vi "input into database.vi"() -> ()   [LabVIEW 2016]
uses:
  controls/db cluster.ctl
  <vilib>/addons/database/Connection.llb/DB Tools Open Connec (String).vi
  <vilib>/Utility/file.llb/Read From Spreadsheet File (string).vi
  <vilib>/addons/database/NI_Database_API.lvlib
panel:
  in  "runnumber":string
  out "output cluster 2":T1
  out "error out":errorcluster
  out "error out 2":errorcluster
  out "element":string="{0.023339,0.023338,0.023336,0.023338,0.023336,0.023336,0.023334\r\n}"
  out "readouts string":string="\r\n1/4/2012 10:09:06 AM\t103752\tWeavCaMB11\tb\tJackson\t0\t3\t50\t1231.000000\tInf\t35.314700\t5.667000\t336.000000\t0.988235\t3599.788248\t31.964787\t6135967.567040\t26573.858939\t1411896.374545\t0.000620\t59.996471\t23532.990455\tNaN\tInf\t0.000000\tNaN\t0.000000\t879579.012026\tNaN\t26573.858939\t0.433083\tNaN\tNaN\tNaN\t7.758172"
  in  "beamline readbacks":T2={"Injector"=[0.023339, 0.023338, 0.023336000000000003, 0.023338, 0.023336000000000003, 0.023336000000000003, 0.023334], "Analyze"=[0.0058, 0.0058, 0.0058, 0.0058, 0.0058, 0.0058, 0.0058], "Switch"=[0.0, 0.0, 0.0, 0.0, 0.0, 0.0, 0.0], "Terminal"=[0.0010328292846679688, 0.0010328292846679688, 0.0013613700866699219, 0.0007047653198242188, 0.0010328292846679688, 0.0010328292846679688, 0.0010328292846679688], "Cathode"=[10.239062309265137, 10.239218711853027, 10.239218711853027, 10.239218711853027, 10.239218711853027, 10.239218711853027, 10.239218711853027]}
  out "db cluster":T3={"startat"="\r\n1/4/2012 10:09:06 AM", "holderid"="103752", "Sample Name"="WeavCaMB11", "type"="b", "User Name"="Jackson", "cycle measured"="0", "position"="3", "estimated ratio"="50", "cycle"="1231.000000", "Transmission"="Inf", "first currents"="35.314700", "runtime"="5.667000", "total rare counts"="336.000000", "livetime"="0.988235", "Rare CPM"="3599.788248", "second current"="31.964787", "17O ratio"="6135967.567040", "17O error"="26573.858939", "Cycle Ratio"="1411896.374545", "cycle error"="0.000620", "interference"="59.996471", "use"="True", "InjSS"="NaN", "He SS"="Inf", "Oaverage"="0.000000", "wheelnumber"="46", "wheel name"="cycle results testdbrunorder.txt", "runnumber"="{0.023339,0.023338,0.023336,0.023338,0.023336,0.023336,0.023334\r\n}", "runletter"="{0.005800,0.005800,0.005800,0.005800,0.005800,0.005800,0.005800\r\n}", "runletter 2"="{0.000000,0.000000,0.000000,0.000000,0.000000,0.000000,0.000000\r\n}"}
  out "name 2":string
  out "name":string
  in  "beamline readbacks 2":T2
  in  "Wheel Number":string
  in  "runletter":string
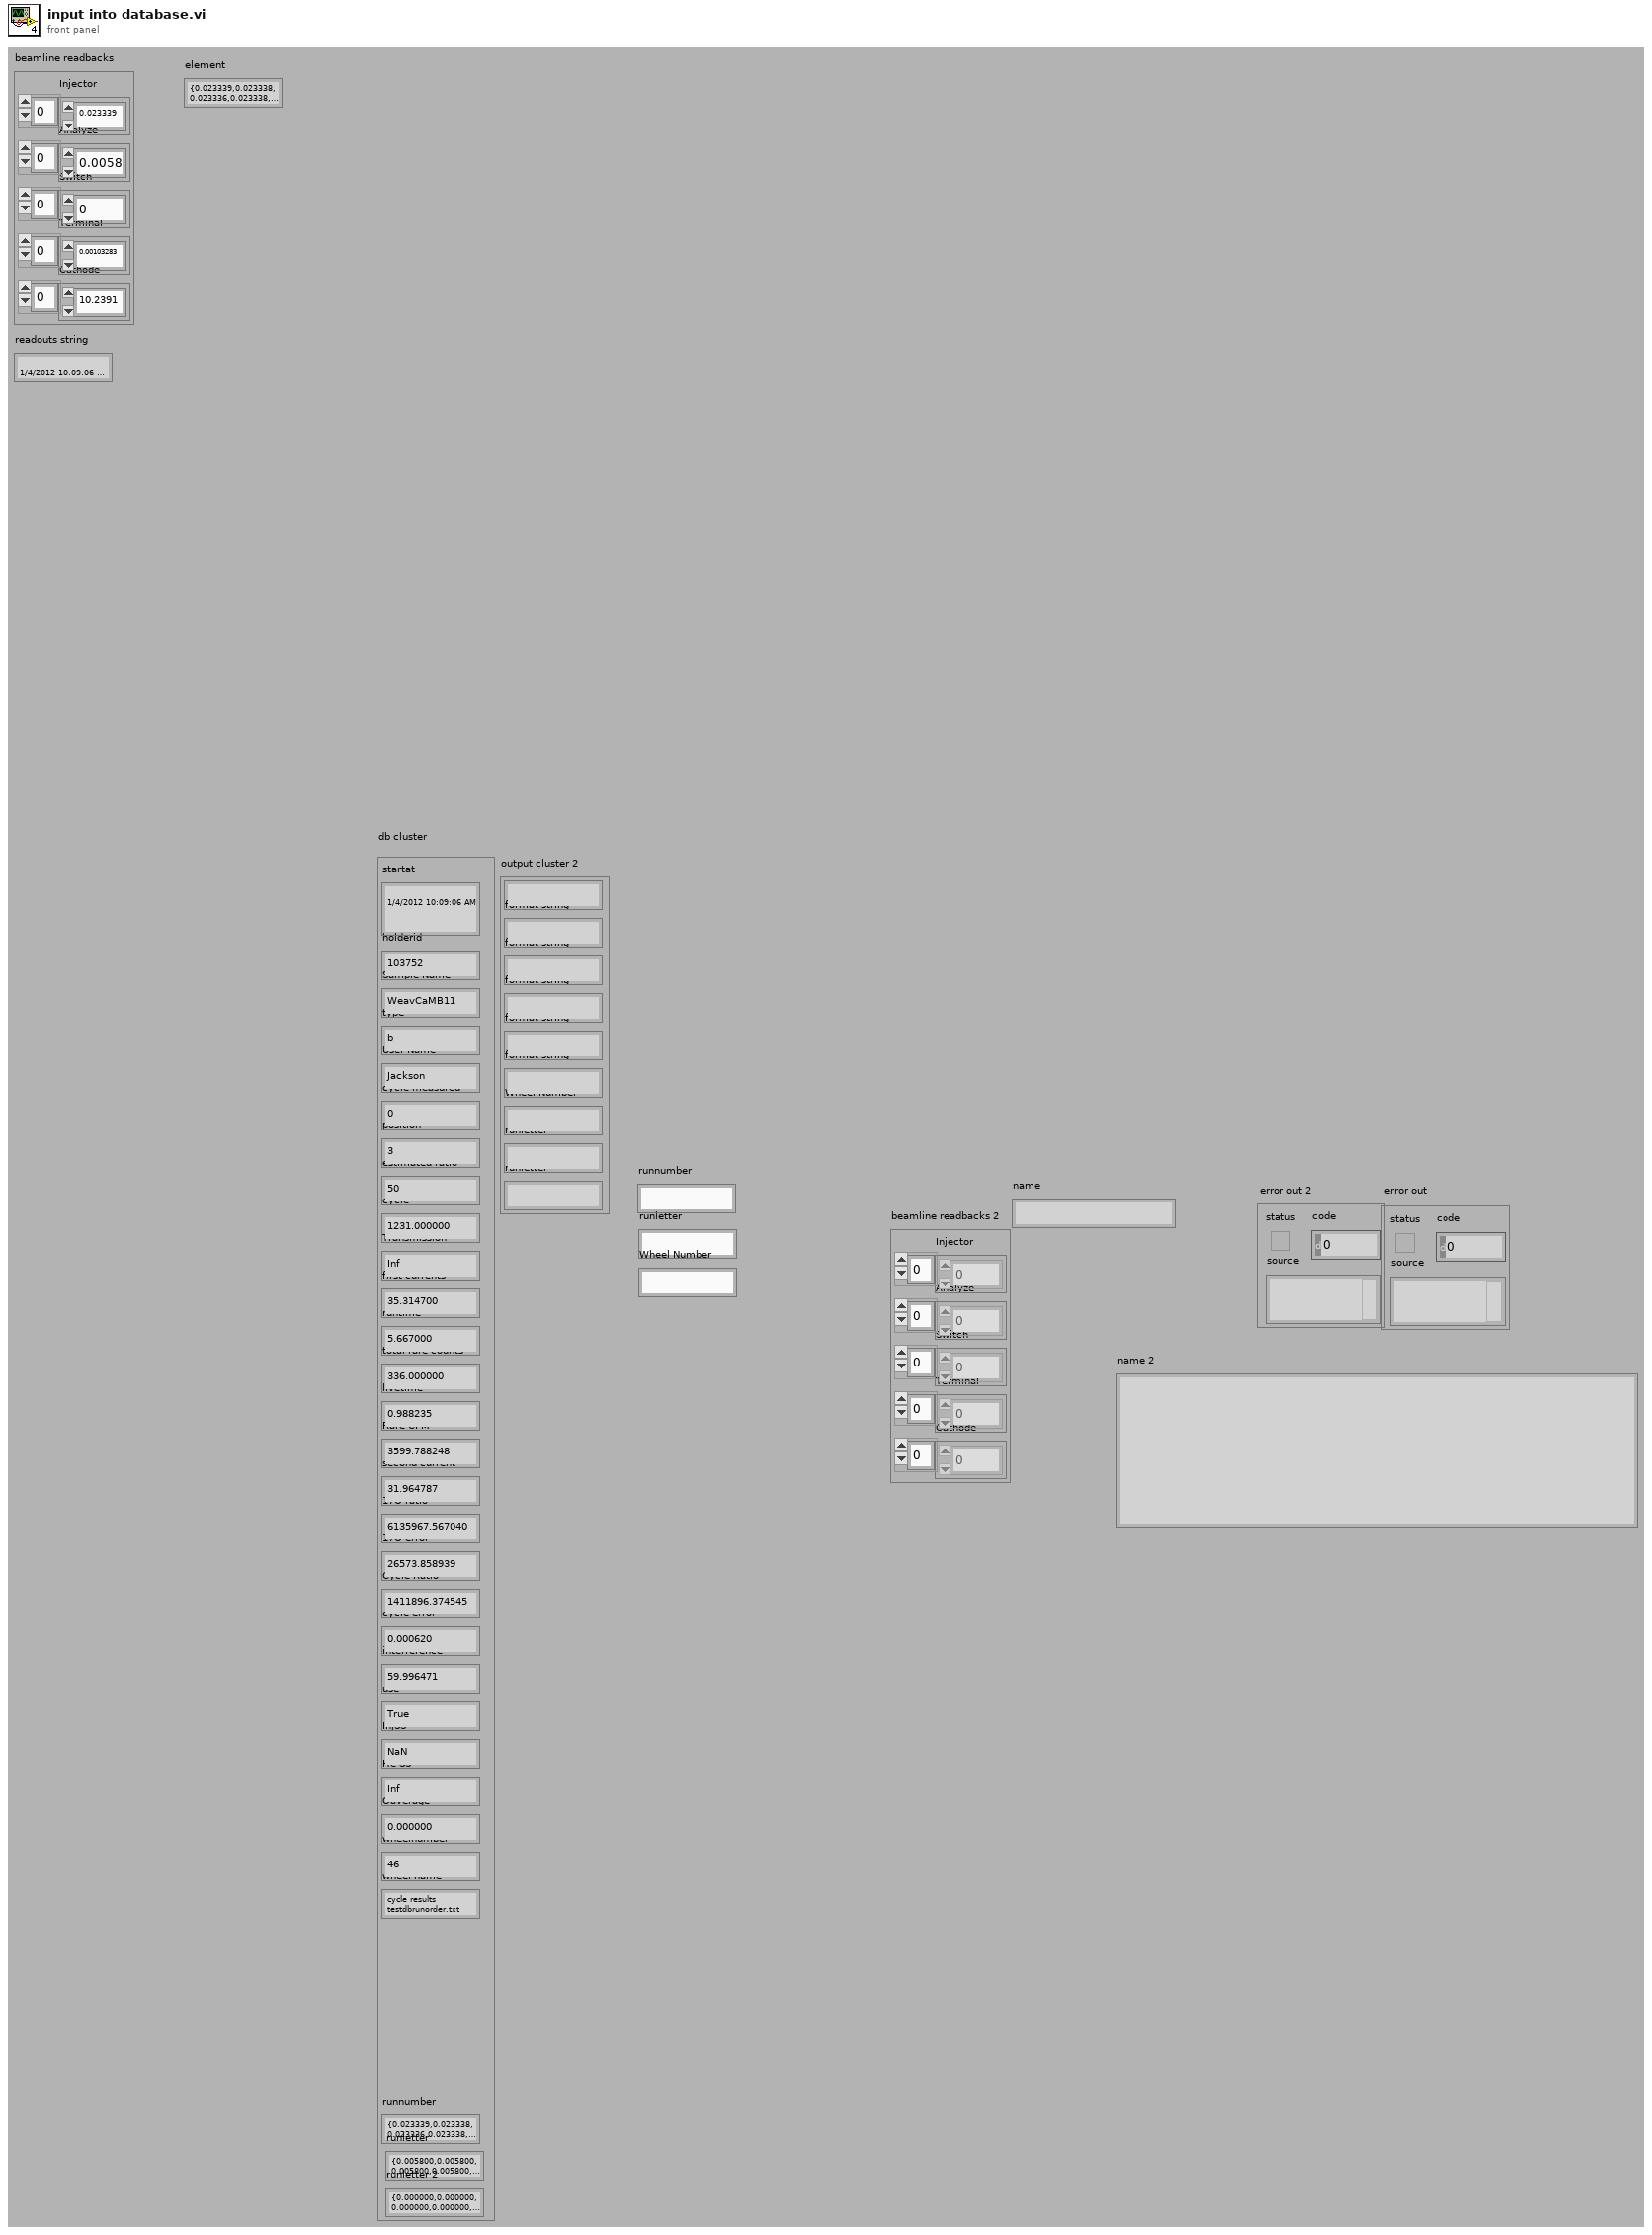
[diagram p1: front panel]
types:
  T1 = cluster{string, "format string":string, "format string":string, "format string":string, "format string":string, "format string":string, "Wheel Number":string, "runletter":string, "runletter":string}
  T2 = cluster{"Injector":dbl[], "Analyze":dbl[], "Switch":dbl[], "Terminal":dbl[], "Cathode":dbl[]}
  T3 = typedef "db cluster.ctl" = cluster{"startat":string, "holderid":string, "Sample Name":string, "type":string, "User Name":string, "cycle measured":string, "position":string, "estimated ratio":string, "cycle":string, "Transmission":string, "first currents":string, "runtime":string, "total rare counts":string, "livetime":string, "Rare CPM":string, "second current":string, "17O ratio":string, "17O error":string, "Cycle Ratio":string, "cycle error":string, "interference":string, "use":string, "InjSS":string, "He SS":string, "Oaverage":string, "wheelnumber":string, "wheel name":string, "runnumber":string, "runletter":string, "runletter 2":string}
  T4 = typedef "NI_Database_API.lvlib/Conn ObjectReference.ctl" = refnum<k1>
  T5 = cluster{"[0]":string, "[1]":string, "[2]":string, "[3]":string, "[4]":string, "[5]":string, "[6]":string, "[7]":string, "[8]":string, "[9]":string, "[10]":string, "[11]":string, "[12]":string, "[13]":string, "[14]":string, "[15]":string, "[16]":string, "[17]":string, "[18]":string, "[19]":string, "[20]":string, "[21]":string, "[22]":string, "[23]":string, "[24]":string, "[25]":string, "[26]":string, "[27]":string, "[28]":string, "[29]":string}
  T6 = cluster{string, "format string":string, "format string":string, "format string":string, "format string":string, "format string":string, "runnumber":string, "runletter":string, "runletter":string}
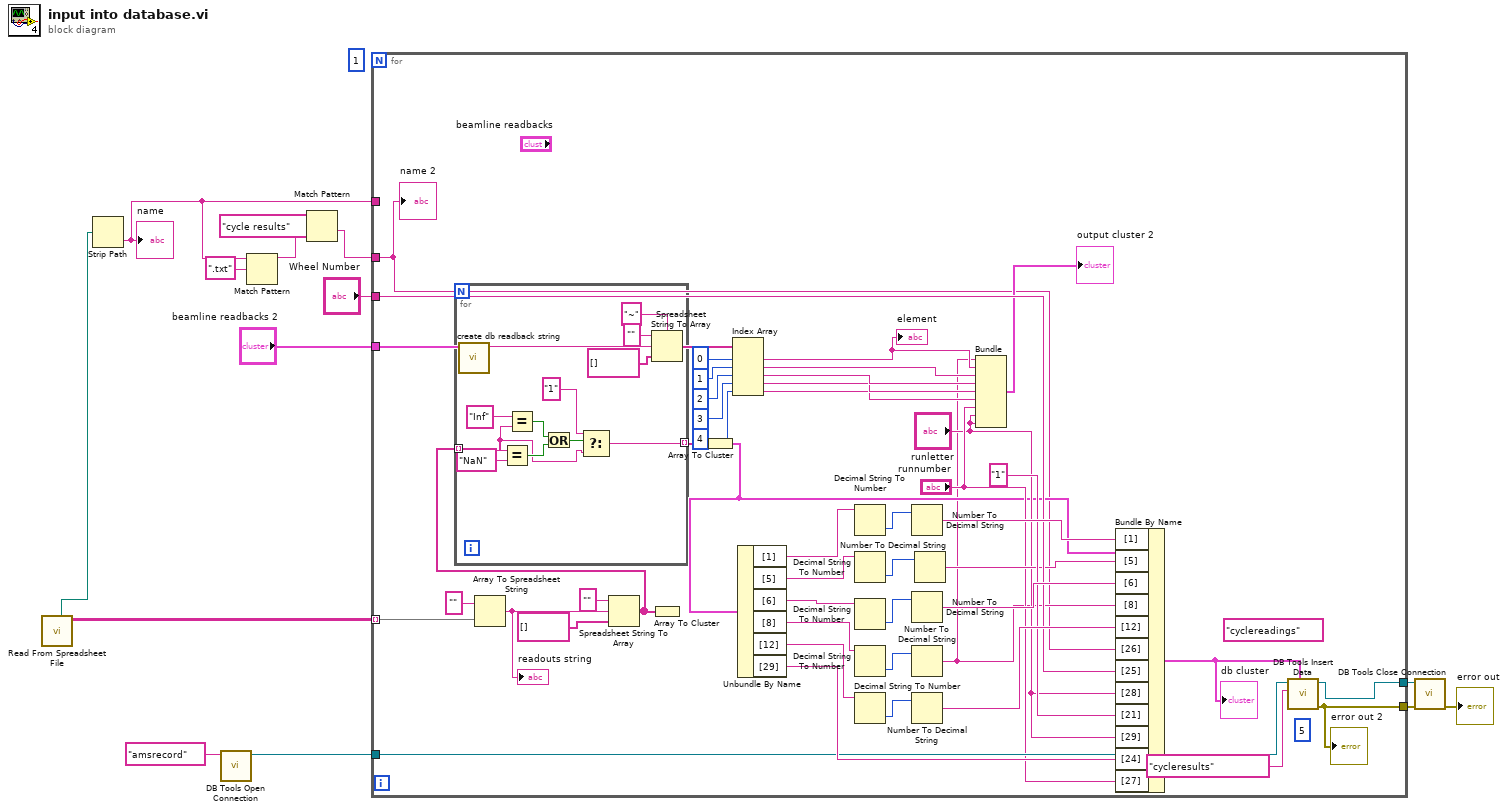
[diagram p0: block diagram]
diagram:
  (unwired) 1
  n1 = call-poly <vilib>:"Read From Spreadsheet File.vi"() -> ("all rows"=w14:string[][], "new file path (Not A Path if cancelled)"=w12:path)  [unwired: 7 in, 3 out]
  n2 = Strip Path(path=w12) -> (name=w9:string)  [unwired: 1 out]
  "name" <- w9
  n3 = call-poly <vilib>:"DB Tools Open Connection.vi"("connection information"="amsrecord") -> ("connection reference"=w7:T4)  [unwired: 7 in, 1 out]
  n4 = Match Pattern(string=w9, regular expression=".txt") -> (before substring=w3:string)  [unwired: 1 in, 3 out]
  n5 = Match Pattern(string=w3, regular expression="cycle results") -> (after substring=w1:string)  [unwired: 1 in, 3 out]
  n6 = for {
    tunnel: w14 -> [w65] mode=indexing
    tunnel: "beamline readbacks 2" -> [w35]
    tunnel: w9 -> [_]
    tunnel: "Wheel Number" -> [w34]
    tunnel: w1 -> [w16]
    tunnel: w7 -> [w32]
    tunnel: [w15] -> w6
    tunnel: [w17] -> w5
    (unwired) "cyclereadings" ("table")
    (unwired) 5 ("index (col)")
    n7 = call "create db readback string.vi"("beamline readbacks"=w35) -> ("arry of readback strings"=w48:string)  [unwired: 9 in, 1 out]
    n8 = Array To Spreadsheet String(array=w65, 3:"" ("format string")) -> (spreadsheet string=w33:string)  [unwired: 1 in]
    "readouts string" <- w33
    n9 = Spreadsheet String To Array(format string="", spreadsheet string=w33, array type (2D Dbl)=string[] []) -> (array=w21:string[])  [unwired: 1 in]
    n10 = for {
      tunnel: w21 -> [w68] mode=indexing
      tunnel: [w66] -> w22 mode=indexing
      n11 = Equal?(x=w68, y="NaN") -> (x = y?=w70:bool)
      n12 = Equal?(x="Inf" ("y"), y=w68) -> (x = y?=w71:bool)
      n13 = Or(x=w71, y=w70) -> (x .or. y?=w69:bool)
      n14 = Select(t="1", s=w69, f=w68) -> (s? t:f=w66:string)
    }
    n15 = Spreadsheet String To Array(delimiter (Tab)="~", format string="", spreadsheet string=w48, array type (2D Dbl)=string[] []) -> (array=w42:string[])
    n16 = Array To Cluster(array=w21) -> ()  [unwired: 1 out]
    n17 = Array To Cluster(array=w22) -> (cluster=w20:T5)
    n18 = Index Array(array=w42, index #1=0 ("disabled index (col)"), index #2=1 ("index (col)"), index #3=2 ("index (col)"), index #4=3 ("index (col)"), index #5=4 ("index (col)")) -> (element #1=w23:string, element #2=w24:string, element #3=w29:string, element #4=w28:string, element #5=w27:string)
    "element" <- w23
    n19 = Unbundle By Name(w20) -> ("[1]"=w50:string, "[5]"=w51:string, "[6]"=w52:string, "[8]"=w56:string, "[12]"=w57:string, "[29]"=w63:string)
    n20 = Decimal String To Number(string=w50) -> (number=w62:i32)  [unwired: 2 in, 1 out]
    n21 = Decimal String To Number(string=w51) -> (number=w61:i32)  [unwired: 2 in, 1 out]
    n22 = Decimal String To Number(string=w52) -> (number=w60:i32)  [unwired: 2 in, 1 out]
    n23 = Decimal String To Number(string=w56) -> (number=w55:i32)  [unwired: 2 in, 1 out]
    n24 = Decimal String To Number(string=w57) -> (number=w58:i32)  [unwired: 2 in, 1 out]
    n25 = Number To Decimal String(number=w62) -> (decimal integer string=w53:string)  [unwired: 1 in]
    n26 = Number To Decimal String(number=w60) -> (decimal integer string=w54:string)  [unwired: 1 in]
    n27 = Number To Decimal String(number=w55) -> (decimal integer string=w19:string)  [unwired: 1 in]
    n28 = Number To Decimal String(number=w58) -> (decimal integer string=w59:string)  [unwired: 1 in]
    n29 = Number To Decimal String(number=w61) -> (decimal integer string=w30:string)  [unwired: 1 in]
    n30 = Bundle(w19, "format string"=w23, "format string"=w24, "format string"=w29, "format string"=w28, "format string"=w27, "runnumber"="runnumber", "runletter"="runletter", "runletter"="runletter") -> (→"output cluster 2":T6)  [unwired: 1 in]
    n31 = Bundle By Name(cluster=w20, "[1]"=w53, "[5]"=w30, "[6]"=w54, "[8]"=w19, "[12]"=w59, "[26]"=w16, "[25]"=w34, "[28]"="runletter", "[21]"="1" ("format string"), "[29]"="runletter", "[24]"=w63, "[27]"="runnumber") -> (w31:T5)
    "db cluster" <- w31
    n32 = call <vilib>:"DB Tools Insert Data.vi"("data"=w31, "table"="cycleresults" ("String"), "connection reference"=w32) -> ("error out"=w15:errorcluster, "connection reference out"=w17:T4)  [unwired: 7 in]
    "error out 2" <- w15
    "name 2" <- w16
  }
  n33 = call <vilib>:"DB Tools Close Connection.vi"("error in (no error)"=w6, "connection reference"=w5) -> ("error out"=→"error out":errorcluster)  [unwired: 5 in]
